vi "Decode Application Message (Raw).vi"(8 "error in (no error)":errorcluster, 10 "PUBLISH":refnum<class "PUBLISH.lvclass">, 11 "Client in":refnum<class "Client.lvclass">) -> (0 "error out":errorcluster, 1 "Payload":u8[](array[numeric]) format="%08b", 2 "Topic":string, 3 "Client out":refnum<class "Client.lvclass">)   [LabVIEW 2013, in "MQTT Client.lvlib" / "Client.lvclass"]
uses:
  Client.lvclass
  <vilib>/LabVIEW Open Source Project/MQTT Control Packets/Control Packets/PUBLISH/PUBLISH.lvclass
  <vilib>/LabVIEW Open Source Project/MQTT Connection/MQTT_Base/Base Class/MQTT_Base.lvclass
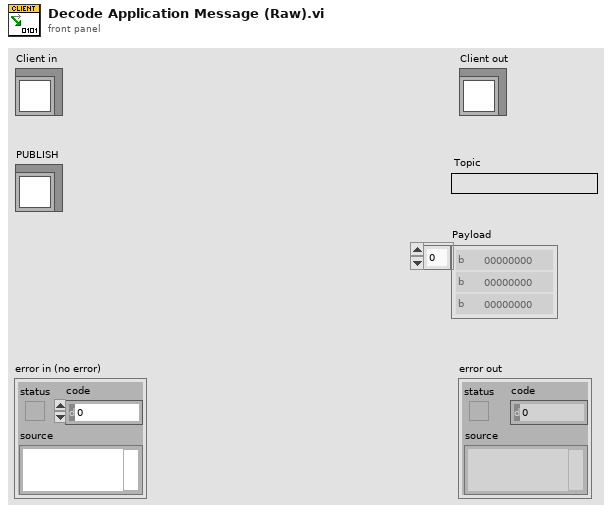
[diagram p1: front panel]
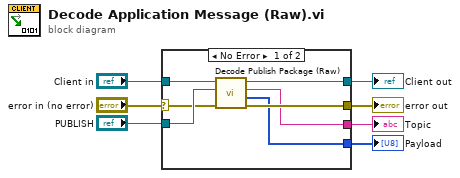
[diagram p0: block diagram]
diagram:
  n1 = case shown="No Error" "error in (no error)" {
    selector: "error in (no error)" -> [w11 w16]
    tunnel: [w10 w16] -> w6
    tunnel: [w13 w15] -> w4
    tunnel: "Client in" -> [w14 w15]
    tunnel: "PUBLISH" -> [w12 _]
    tunnel: [w9 _] -> w2
    tunnel: [w8 _] -> w1
    frame No Error {
      n2 = call <vilib>:"Decode Publish Package (Raw).vi"("error in (no error)"=w11, "PUBLISH"=w12, "MQTT_Base in"=w14) -> ("error out"=w10:errorcluster, "Payload"=w9:u8[], "Topic"=w8:string, "MQTT_Base out"=w13:refnum<class "Client.lvclass">)  [unwired: 5 in]
    }
    frame Error {
    }
  }
  "error out" <- w6
  "Client out" <- w4
  "Topic" <- w1
  "Payload" <- w2
